vi "Get Msgs.vi"(11 "Base Actor in":refnum<class "Base Actor.lvclass">) -> (2 "Msgs":T1)   [LabVIEW 2020, in "jettl.lvlib" / "Actor.lvlib" / "Base Actor.lvclass"]
uses:
  Base Actor.lvclass
  Msgs.ctl
  Msg/Msg.lvclass
  Base Actor.lvclass/Base Actor.ctl
  Actor.lvlib
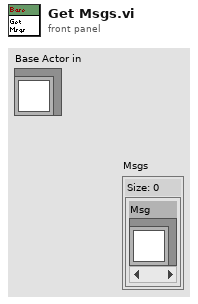
[diagram p1: front panel]
types:
  T1 = typedef "jettl.lvlib/Actor.lvlib/Msgs.ctl" = set{refnum<class "Msg.lvclass">}
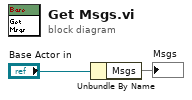
[diagram p0: block diagram]
diagram:
  n1 = Unbundle By Name("Base Actor in") -> ("Msgs"=→"Msgs":T1)
